vi "GetParameterValueString.vi"(8 "error in (no error)":errorcluster, 11 "Parameter in":refnum<class "Parameter.lvclass">) -> (0 "error out":errorcluster, 2 "Value":string, 3 "Parameter out":refnum<class "Parameter.lvclass">)   [LabVIEW 2023, in "Easy.SequenceManagerLabVIEW.lvlib" / "Parameter.lvclass"]
uses:
  Parameter.lvclass
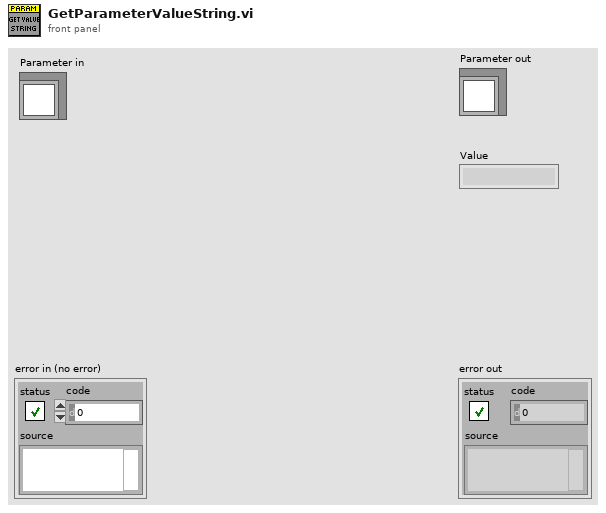
[diagram p1: front panel]
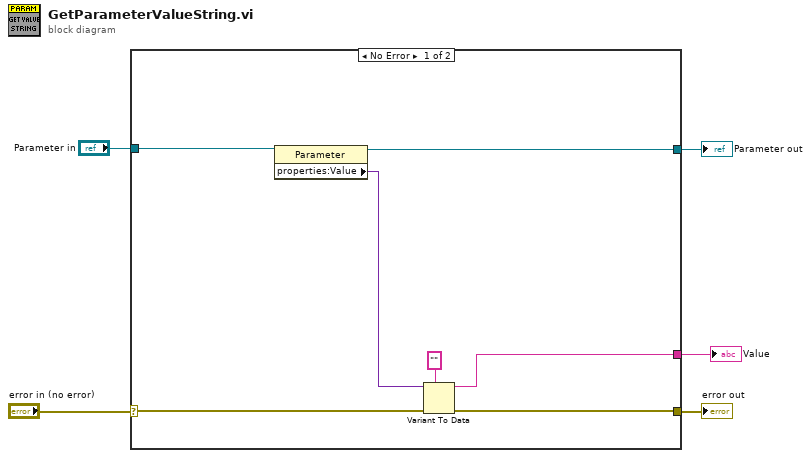
[diagram p0: block diagram]
diagram:
  n1 = case shown="No Error" "error in (no error)" {
    selector: "error in (no error)" -> [w12 w14]
    tunnel: [w8 w14] -> w4
    tunnel: "Parameter in" -> [w6 w13]
    tunnel: [w9 _] -> w2
    tunnel: [w7 w13] -> w1
    frame No Error {
      n2 = property class="Parameter"(reference=w6) -> (reference out=w7:refnum<class "Parameter.lvclass">, "properties:Value"=w10:variant)  [unwired: 1 in, 1 out]
      n3 = Variant To Data(error in=w12, type="", Variant=w10) -> (data=w9:string, error out=w8:errorcluster)
    }
    frame Error {
    }
  }
  "error out" <- w4
  "Parameter out" <- w1
  "Value" <- w2
